vi "run_parallel.vi"   [LabVIEW 2023]
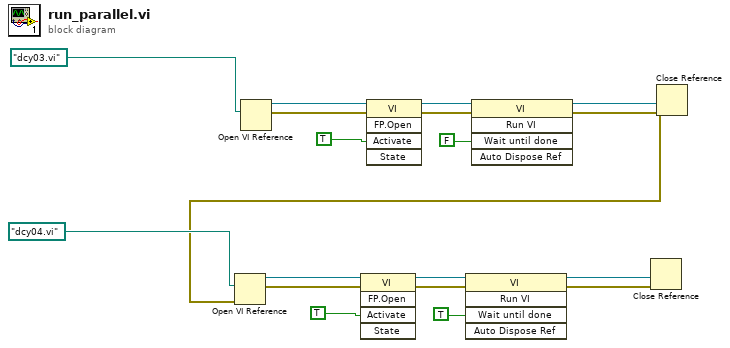
[diagram p0: block diagram]
diagram:
  n1 = Open VI Reference(vi path=path "dcy03.vi") -> (vi reference=w18:refnum<vi>, error out=w17:errorcluster)  [unwired: 5 in]
  n2 = invoke class="VI" method="FP.Open"(reference=w18, error in=w17, "Activate"=TRUE) -> (reference out=w15:refnum<vi>, error out=w14:errorcluster)  [unwired: 2 in, 3 out]
  n3 = invoke class="VI" method="Run VI"(reference=w15, error in=w14, "Wait until done"=FALSE) -> (reference out=w12:refnum<vi>, error out=w11:errorcluster)  [unwired: 2 in, 3 out]
  n4 = Close Reference(reference=w12, error in (no error)=w11) -> (error out=w1:errorcluster)
  n5 = Open VI Reference(vi path=path "dcy04.vi", error in (no error)=w1) -> (vi reference=w9:refnum<vi>, error out=w8:errorcluster)  [unwired: 4 in]
  n6 = invoke class="VI" method="FP.Open"(reference=w9, error in=w8, "Activate"=TRUE) -> (reference out=w6:refnum<vi>, error out=w5:errorcluster)  [unwired: 2 in, 3 out]
  n7 = invoke class="VI" method="Run VI"(reference=w6, error in=w5, "Wait until done"=TRUE) -> (reference out=w3:refnum<vi>, error out=w2:errorcluster)  [unwired: 2 in, 3 out]
  n8 = Close Reference(reference=w3, error in (no error)=w2) -> ()  [unwired: 1 out]
